vi "Set Trigger Sense Div.vi"(10 "y_scale":dbl, 11 "sense":dbl) -> ()   [LabVIEW 2021, in "vmmso.lvlib"]
doc: "DLL_API void WINAPI SetTriggerSenseDiv(double sense, double y_scale);"
uses:
  vmmso.lvlib
  vmmso.dll
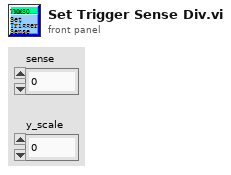
[diagram p1: front panel]
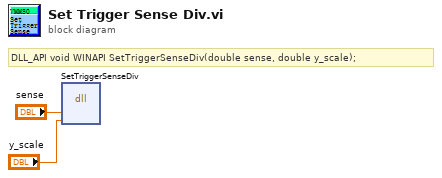
[diagram p0: block diagram]
diagram:
  # "DLL_API void WINAPI SetTriggerSenseDiv(double sense, double y_scale);"
  n1 = dll-call lib="D:/labviewdemo/LabviewDemo 21/vmmso/vmmso.*" fn="SetTriggerSenseDiv"("sense"="sense", "y_scale"="y_scale") -> ()  [unwired: 6 in, 2 out]
